vi "Test SenseHat Write Read Raw.vi"() -> ()   [LabVIEW 2020]
uses:
  <vilib>/MakerHub/LINX/LMH-LINX.lvlib
  src/RPI.SenseHat.Display/Classes/SenseHat.Display/RPI.SenseHat.Display.lvclass
  <vilib>/MakerHub/LINX/Public/Utilities/Open Local.vi
panel:
  out "Data":u8[](array[numeric])
  out "Device Name":string
  out "Error Out":errorcluster
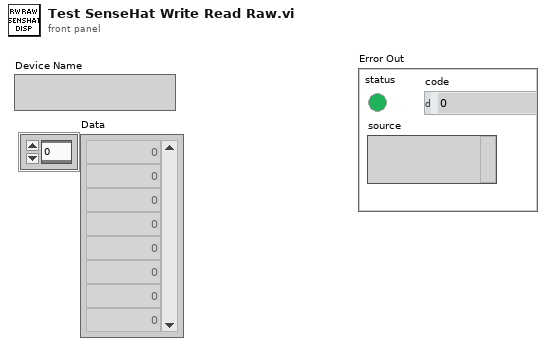
[diagram p1: front panel]
types:
  T1 = typedef "LMH-LINX.lvlib/LINX Ref.ctl" = cluster{"IO":T2, "Interface":T3, "LINX Device Config":T4}
  T2 = typedef "LMH-LINX.lvlib/Platform.ctl" = enum16{"Remote", "Local"}
  T3 = typedef "LMH-LINX.lvlib/Interface.ctl" = enum16{"Serial", "TCP"}
  T4 = typedef "LMH-LINX.lvlib/Device.lvlib/LINX Device Config.ctl" = cluster{"Interface":T3, "COM Port":refnum<visa-resource-name>, "TCP Configuration":T5, "Device Family":u8, "Device ID":u8, "Device Name":string, "TCP Ref":refnum<k5>, "Channels":T6}
  T5 = typedef "LMH-LINX.lvlib/Device.lvlib/TCP Config.ctl" = cluster{"IP Address":string, "Port":u16}
  T6 = typedef "LMH-LINX.lvlib/Channels.ctl" = cluster{"DI":u8[], "DO":u8[], "AI":u8[], "AO":u8[], "PWM":u8[], "QE":u8[], "UART":u8[], "I2C 2":u8[], "SPI":u8[], "CAN":u8[], "Servo":u8[], "AI Ref (V)":dbl, "AI Resolution (Bits)":u8, "AO Ref (V)":dbl, "AO Resolution (Bits)":u8}
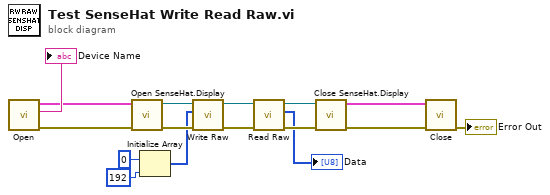
[diagram p0: block diagram]
diagram:
  n1 = call-poly <vilib>:"Open.vi"() -> ("Error Out"=w14:errorcluster, "Device Name"=→"Device Name":string, "LINX Resource"=w7:T1)  [unwired: 9 in]
  n2 = call "Open SenseHat.Display.vi"("error in (no error)"=w14, "LINX Resource"=w7) -> ("error out"=w13:errorcluster, "senseHatDisplay out"=w12:refnum<class "RPI.SenseHat.Display.lvclass">)  [unwired: 8 in]
  n3 = Initialize Array(u8 0 ("element"), 192 ("dimension size")) -> (w2:u8[])
  n4 = call "Write Raw.vi"("error in (no error)"=w13, "Data"=w2, "senseHatDisplay in"=w12) -> ("error out"=w6:errorcluster, "senseHatDisplay out"=w5:refnum<class "RPI.SenseHat.Display.lvclass">)  [unwired: 7 in]
  n5 = call "Read Raw.vi"("error in (no error)"=w6, "senseHatDisplay in"=w5) -> ("error out"=w10:errorcluster, "Data"=→"Data":u8[], "senseHatDisplay out"=w11:refnum<class "RPI.SenseHat.Display.lvclass">)  [unwired: 7 in]
  n6 = call "Close SenseHat.Display.vi"("error in (no error)"=w10, "senseHatDisplay in"=w11) -> ("error out"=w15:errorcluster, "LINX Resource"=w16:T1)  [unwired: 8 in]
  n7 = call <vilib>:"Close.vi"("Error In"=w15, "LINX Resource"=w16) -> ("Error Out"=→"Error Out":errorcluster)  [unwired: 9 in]
